vi "Write Instrument Name.vi"(8 "error in (no error)":errorcluster, 10 "Instrument Name":string, 11 "Dynamic Instrument in":refnum<class "Dynamic Instrument.lvclass">) -> (0 "error out":errorcluster, 3 "Dynamic Instrument out":refnum<class "Dynamic Instrument.lvclass">)   [LabVIEW 2016, in "Dynamic Instrument.lvlib" / "Dynamic Instrument.lvclass"]
uses:
  Dynamic Instrument.lvclass
  Dynamic Instrument.lvclass/Dynamic Instrument.ctl
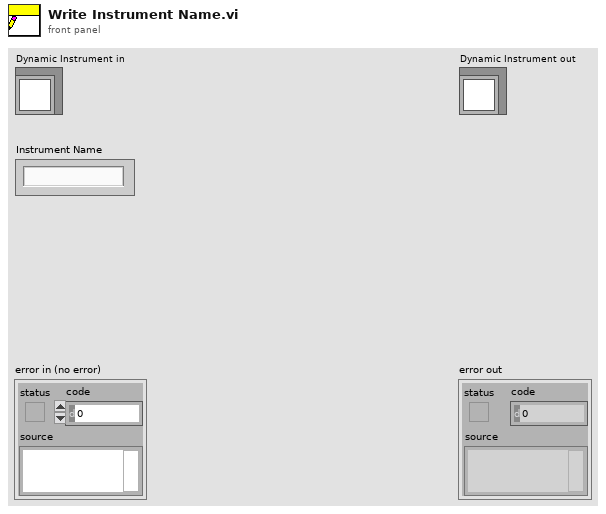
[diagram p1: front panel]
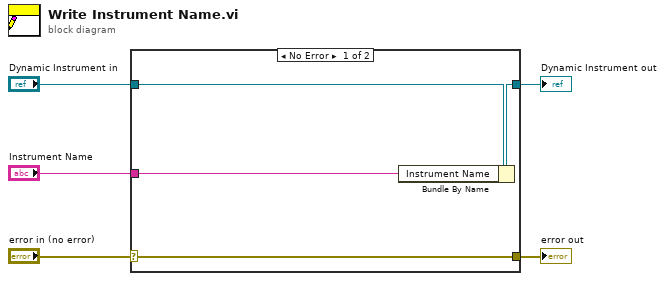
[diagram p0: block diagram]
diagram:
  n1 = case shown="No Error" "error in (no error)" {
    selector: "error in (no error)" -> [w9 w10]
    tunnel: [w9 w10] -> w4
    tunnel: [w7 w11] -> w2
    tunnel: "Dynamic Instrument in" -> [w8 w11]
    tunnel: "Instrument Name" -> [w6 _]
    frame No Error {
      n2 = Bundle By Name(cluster=w8, "Instrument Name"=w6) -> (w7:refnum<class "Dynamic Instrument.lvclass">)
    }
    frame Error {
    }
  }
  "error out" <- w4
  "Dynamic Instrument out" <- w2
